vi "PRUEBA_NEO_I.vi"() -> ()   [LabVIEW 2025]
panel:
  out "error out":errorcluster
  in  "stop":bool
  in  "Color Box":u32(colorbox)
  in  "No. NeoPixel":u8=1 max=2
  in  "VISA resource name":refnum<visa-resource-name>
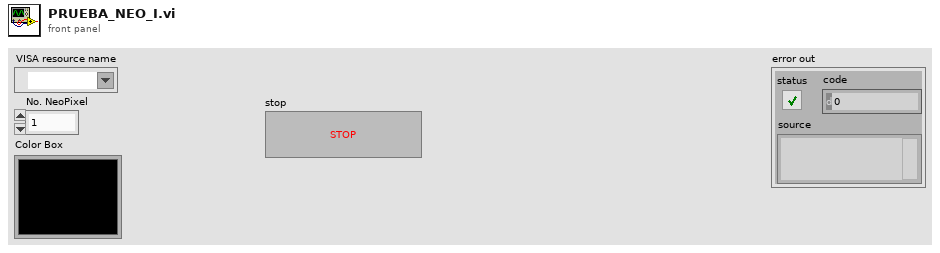
[diagram p1: front panel]
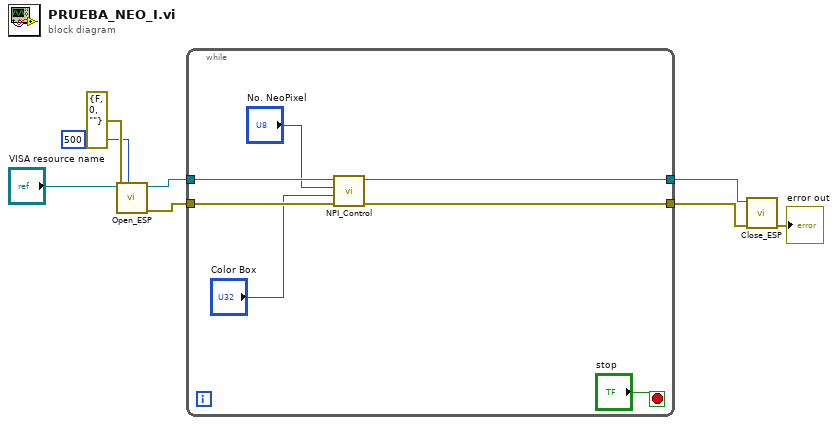
[diagram p0: block diagram]
diagram:
  n1 = call "Open_ESP.vi"("timeout (10sec)"=u32 500, "error in (no error)"=errorcluster {"status"=FALSE, "code"=0, "source"=""}, "VISA resource name"="VISA resource name") -> ("error out"=w3:errorcluster, "VISA resource name out"=w8:refnum<visa-resource-name>)  [unwired: 7 in]
  n2 = while {
    tunnel: w3 -> [w12]
    tunnel: [w14] -> w5
    tunnel: w8 -> [w15]
    tunnel: [w13] -> w4
    stop <- "stop" stop-if-true
    n3 = call "NPI_Control.vi"("error in (no error)"=w12, "Color Box"="Color Box", "No. NeoPixel"="No. NeoPixel", "VISA resource name"=w15) -> ("error out"=w14:errorcluster, "VISA resource name out"=w13:refnum<visa-resource-name>)  [unwired: 6 in]
  }
  n4 = call "Close_ESP.vi"("error in (no error)"=w5, "VISA resource name"=w4) -> ("error out"=→"error out":errorcluster)  [unwired: 9 in]
